vi "Build Socket Mask.vi"(0 "Dev Mask (All)":bool[](array[boolean])=[TRUE, TRUE, TRUE, TRUE, TRUE, TRUE]) -> (4 "Socket Mask [U32]":u32 format="%06x")   [LabVIEW 2017, in "Host SRL.lvlib"]
uses:
  Host SRL.lvlib
panel:
  # "Dev 01"
  # "Dev 02"
  # "Dev 03"
  # "Dev 04"
  # "Dev 05"
  # "Dev 06"
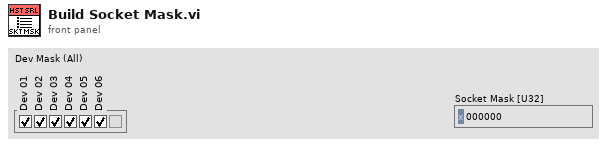
[diagram p1: front panel]
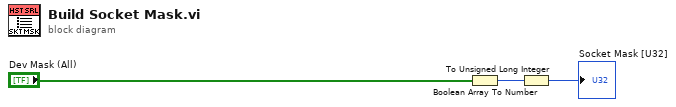
[diagram p0: block diagram]
diagram:
  n1 = Boolean Array To Number(Boolean array="Dev Mask (All)") -> (number=w3:u64)
  n2 = To Unsigned Long Integer(number=w3) -> (unsigned 32bit integer=→"Socket Mask [U32]":u32)
